vi "Explore.vi"(8 "error in (no error)":errorcluster, 11 "file path":path) -> (0 "error out":errorcluster)   [LabVIEW 2017]
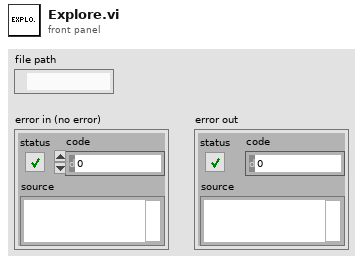
[diagram p1: front panel]
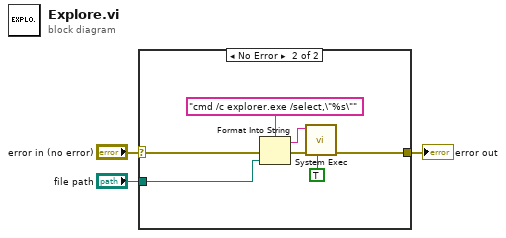
[diagram p0: block diagram]
diagram:
  n1 = case shown="No Error" "error in (no error)" {
    selector: "error in (no error)" -> [w4 w5]
    tunnel: "file path" -> [_ w8]
    tunnel: [w4 w6] -> w1
    frame Error {
    }
    frame No Error {
      n2 = Format Into String(format string="cmd /c explorer.exe /select,\"%s\"", error in=w5, w8) -> (resulting string=w10:string, error out=w7:errorcluster)  [unwired: 1 in]
      n3 = call <vilib>:"System Exec.vi"("run minimized? (F)"=TRUE, "error in (no error)"=w7, "command line"=w10) -> ("error out"=w6:errorcluster)  [unwired: 5 in, 3 out]
    }
  }
  "error out" <- w1
